vi "Configure the Function on 1st Display .vi"(5 "Manual Range":dbl format="%#.9e", 7 "Enable Auto Range":bool=TRUE, 8 "error in":errorcluster, 9 "Type for Temperature":u8(ring) items=["J Type", "K Type", "T Type"], 10 "Function":u8(ring) items=["DC Voltage", "AC Voltage", "DC+AC Voltage", "DC Current", "AC Current", "DC+AC Current", "2-Wire Resistance", "Frequency", "Period", "Continuity", "Diode", "Temperature", "Capacitance"], 11 "VISA resource name":refnum<visa-resource-name>) -> (0 "error out":errorcluster, 3 "VISA resource name out":refnum<visa-resource-name>)   [LabVIEW 2021, in "DMM4.lvlib"]
uses:
  DMM4.lvlib
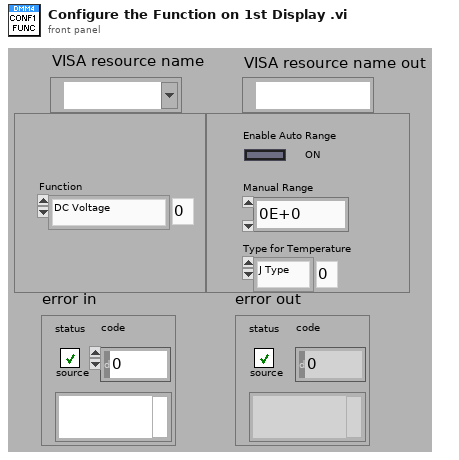
[diagram p1: front panel]
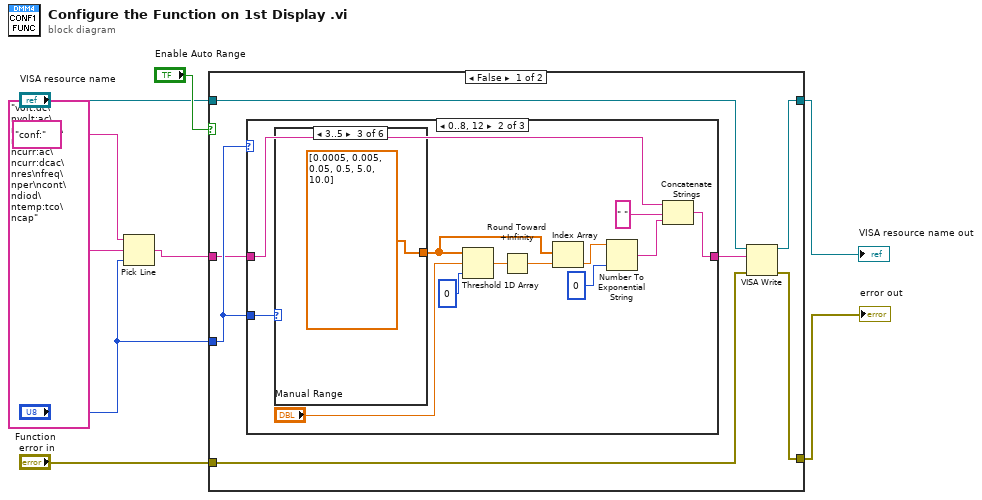
[diagram p0: block diagram]
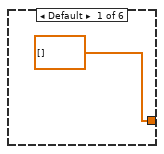
[diagram p3: hidden frame]
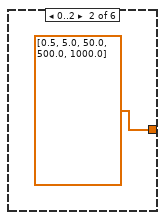
[diagram p4: hidden frame]
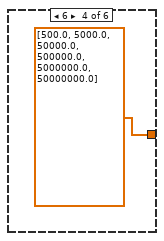
[diagram p5: hidden frame]
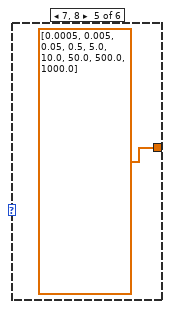
[diagram p6: hidden frame]
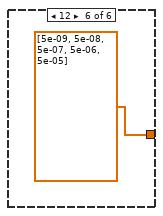
[diagram p7: hidden frame]
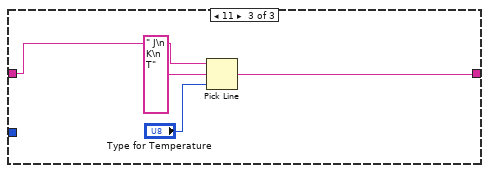
[diagram p8: hidden frame]
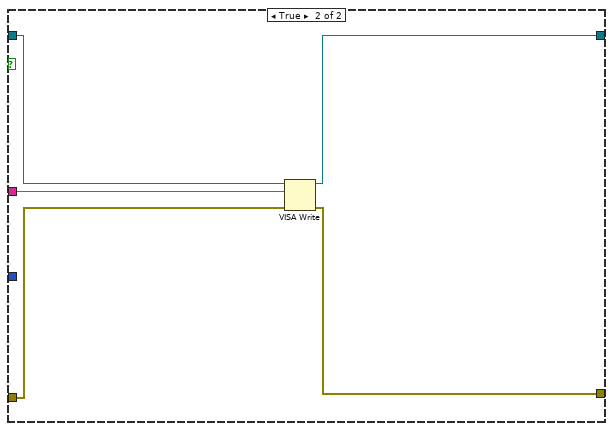
[diagram p9: hidden frame]
diagram:
  n1 = Pick Line(string ("")="conf:", multi-line string="volt:dc\nvolt:ac\nvolt:dcac\ncurr:dc\ncurr:ac\ncurr:dcac\nres\nfreq\nper\ncont\ndiod\ntemp:tco\ncap", line index="Function") -> (output string=w5:string)
  n2 = case shown="False" "Enable Auto Range" {
    tunnel: "Function" -> [w16 _]
    tunnel: w5 -> [w15 w44]
    tunnel: "VISA resource name" -> [w13 w43]
    tunnel: "error in" -> [w12 w42]
    tunnel: [w11 w41] -> w2
    tunnel: [w10 w40] -> w1
    frame False {
      n3 = case shown="0..8, 12" w16 {
        tunnel: w16 -> [_ w18 _]
        tunnel: w15 -> [w17 w20 w36]
        tunnel: [w17 w19 w37] -> w14
        frame Default {
        }
        frame 0..8, 12 {
          n4 = case shown="3..5" w18 {
            tunnel: [dbl[] [] dbl[] [0.5, 5.0, 50.0, 500.0, 1000.0] dbl[] [0.0005, 0.005, 0.05, 0.5, 5.0, 10.0] dbl[] [500.0, 5000.0, 50000.0, 500000.0, 5000000.0, 50000000.0] dbl[] [0.0005, 0.005, 0.05, 0.5, 5.0, 10.0, 50.0, 500.0, 1000.0] dbl[] [5e-09, 5e-08, 5e-07, 5e-06, 5e-05]] -> w25
            frame Default {
            }
            frame 0..2 {
            }
            frame 3..5 {
            }
            frame 6 {
            }
            frame 7, 8 {
            }
            frame 12 {
            }
          }
          n5 = Threshold 1D Array(1:0 ("start index (0)"), 2:"Manual Range", 3:w25) -> (0:w27:dbl)
          n6 = Round Toward +Infinity(x=w27) -> (ceil(x): smallest int >= x=w26:dbl)
          n7 = Index Array(array=w25, index=w26) -> (element=w24:dbl)
          n8 = Number To Exponential String(number=w24, precision (6)=i16 0) -> (E-format string=w21:string)  [unwired: 2 in]
          n9 = Concatenate Strings(w20, " " ("string"), w21) -> (w19:string)
        }
        frame 11 {
          n10 = Pick Line(string ("")=w36, multi-line string=" J\n K\n T", line index="Type for Temperature") -> (output string=w37:string)
        }
      }
      n11 = VISA Write(VISA resource name=w13, write buffer=w14, error in (no error)=w12) -> (VISA resource name out=w11:refnum<visa-resource-name>, error out=w10:errorcluster)  [unwired: 1 out]
    }
    frame True {
      n12 = VISA Write(VISA resource name=w43, write buffer=w44, error in (no error)=w42) -> (VISA resource name out=w41:refnum<visa-resource-name>, error out=w40:errorcluster)  [unwired: 1 out]
    }
  }
  "VISA resource name out" <- w2
  "error out" <- w1
